vi "Demo UI Orientation.vi"(8 "error in (no error)":errorcluster) -> (0 "error out":errorcluster)   [LabVIEW 2011]
uses:
  VIremote.llb/VIremoteEvent.ctl
  VIremote.llb/VIremoteFunction.ctl
  VIremote.llb/VIremoteStatus.ctl
panel:
  out "Hide":bool
  out "Orientation":T1=enum."Portrait"
  in  "VIremoteEvent":T1=enum."Connection Closed"
  # "Rotate your Device!"
  # "If you have locked your device in one orientation this demo will not work."
  # "This VIs orientation is Landscape"
  # "Portrait"
  # "This VIs orientation is Landscape"
  # "Portrait"
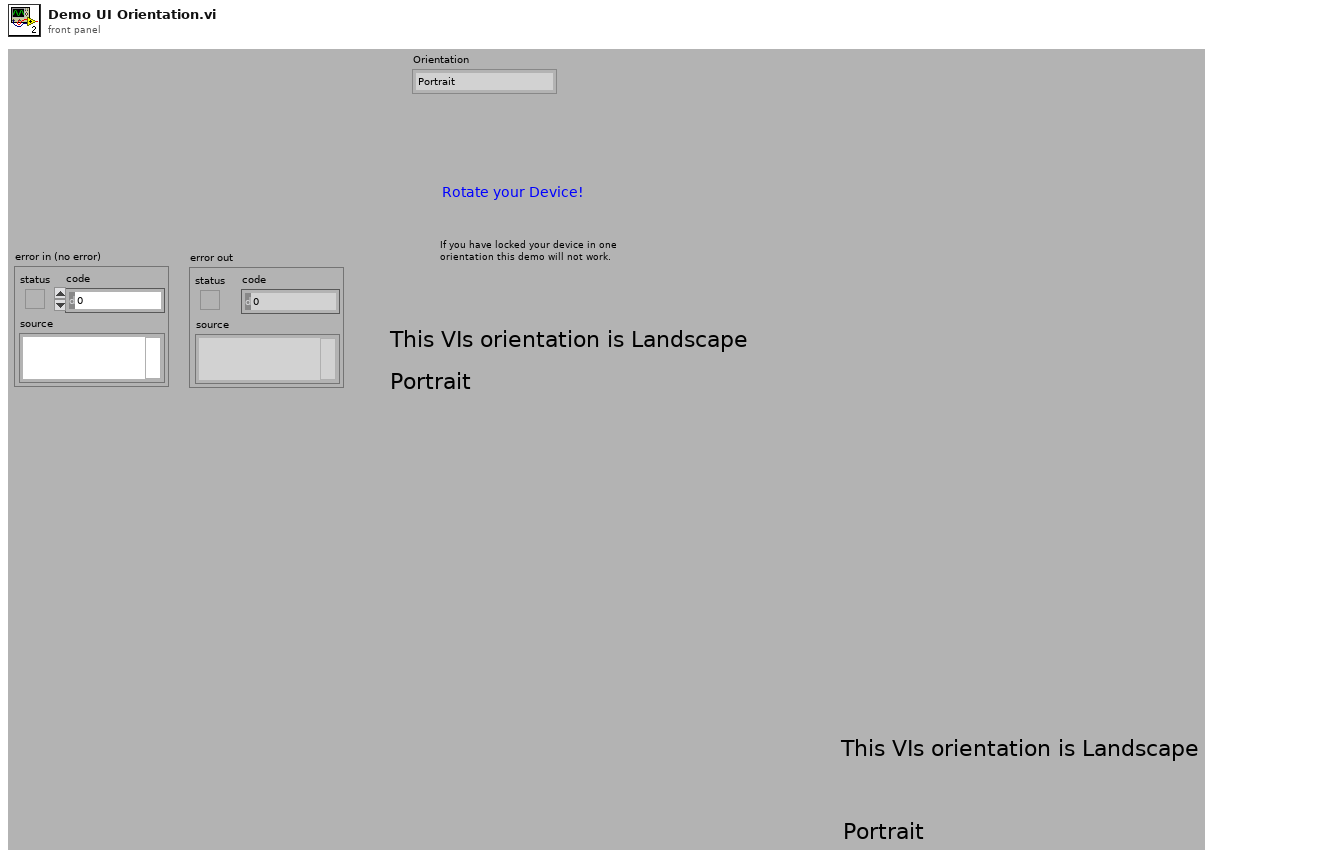
[diagram p1: front panel]
types:
  T1 = typedef "VIremoteEvent.ctl" = enum16{"No Event", "Connection Closed", "Navigate Back", "Enter Background", "Enter Foreground", "Portrait", "Portrait Upside Down", "Landscape Left", "Landscape Right"}
  T2 = typedef "VIremoteStatus.ctl" = enum16{"Connected BOOL", "Number of connections DBL", "VIremoteController ver.", "VIremote ver. DBL", "Screen width DBL", "Screen height DBL", "Current navigation bar height DBL", "Current UI orientation", "Background supported BOOL", "Background state BOOL", "Device UI idiom (0=phone,1=iPad) DBL", "Device name", "Device unique id", "Device system ver.", "Device model", "Device HW model"}
  T3 = typedef "VIremoteFunction.ctl" = enum16{"Do nothing", "Stop controller", "Close this connection", "Show info panel", "Set VI to control", "Set Accelerometer freq (Hz)", "Show Alert message", "Start Sound Input", "Stop Sound Input", "Set Volume (0-100)", "Set sound output Speaker", "Set sound output Receiver", "Play Sound", "Repeat Sound", "Stop Sound", "Pause Sound", "Resume Sound", "Set panel width of caller (320 or 480)", "Set Panel Size to Portrait", "Set Panel Size to Landscape", "Set Panel Size as Current Orientation", "Allow all UI Orientations", "Send user notification", "Disable Scrolling", "Normal Scrolling", "Page Scrolling", "Set Scroll Offset", "Page Indicator Position"}
  T4 = typedef "VIremotePreferences.ctl" = cluster{"Set (must be true)":bool, "allowed UI orientations":cluster{"Portrait":bool, "PortraitUpsideDown":bool, "LandscapeLeft":bool, "LandscapeRight":bool}}
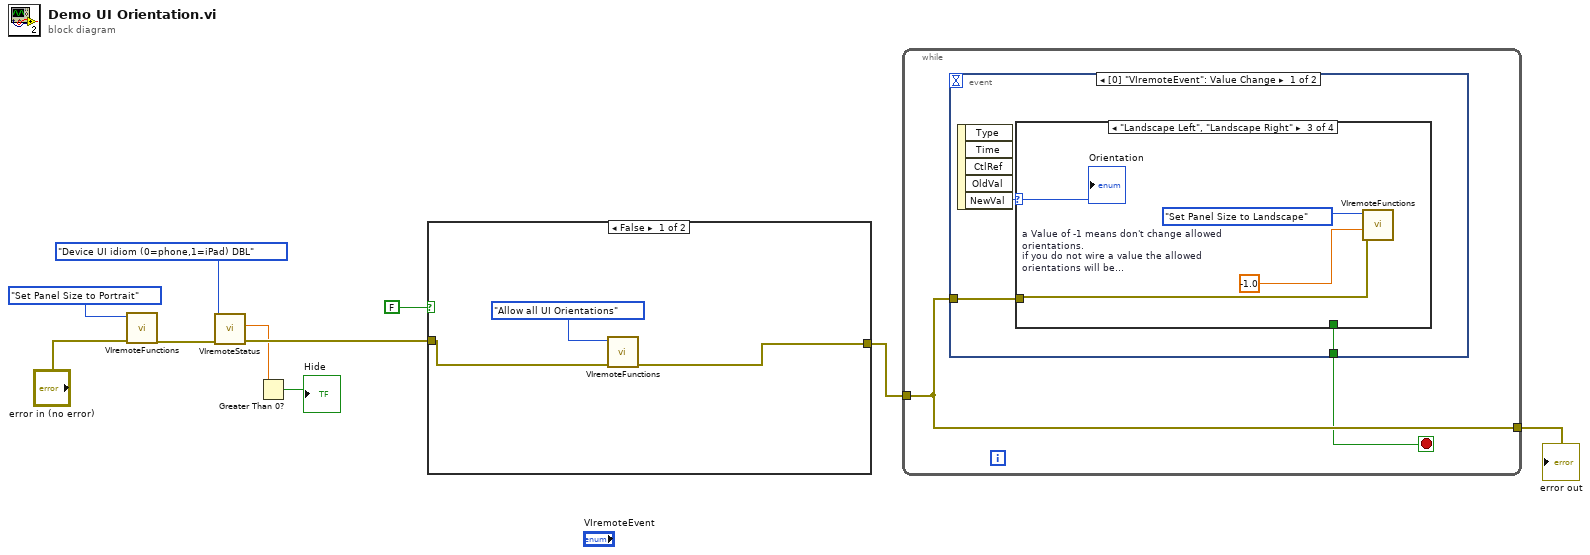
[diagram p0: block diagram]
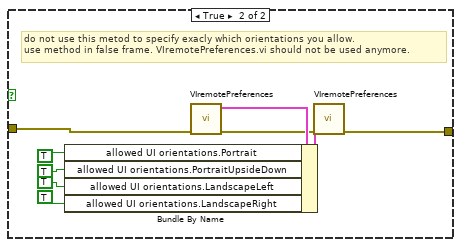
[diagram p2: hidden frame]
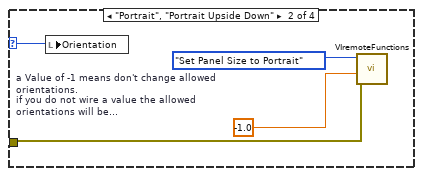
[diagram p4: hidden frame]
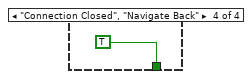
[diagram p5: hidden frame]
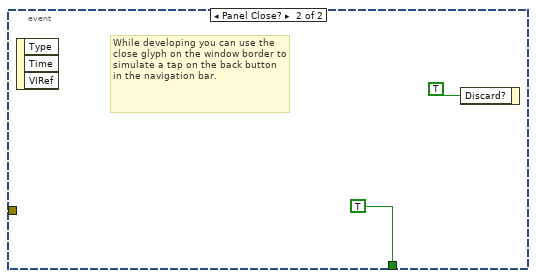
[diagram p6: hidden frame]
diagram:
  n1 = call "VIremoteFunctions.vi"("error in (no error)"="error in (no error)", "Function"=VIremoteFunction."Set Panel Size to Portrait") -> ("error out"=w5:errorcluster)  [unwired: 4 in, 5 out]
  n2 = call "VIremoteStatus.vi"("error in (no error)"=w5, "Status item"=VIremoteStatus."Device UI idiom (0=phone,1=iPad) DBL") -> ("error out"=w4:errorcluster, "DBL"=w2:dbl)  [unwired: 1 in, 7 out]
  n3 = Greater Than 0?(x=w2) -> (x > 0?=→"Hide":bool)
  n4 = case shown="False" FALSE {
    tunnel: [w12 w15] -> w10
    tunnel: w4 -> [w11 w14]
    frame False {
      n5 = call "VIremoteFunctions.vi"("error in (no error)"=w11, "Function"=VIremoteFunction."Allow all UI Orientations") -> ("error out"=w12:errorcluster)  [unwired: 4 in, 5 out]
    }
    frame True {
      # "do not use this metod to specify exacly which orientations you allow.\nuse method in false frame. VIremotePreferences.vi should not be used anymore."
      n6 = call "VIremotePreferences.vi"("error in (no error)"=w14) -> ("error out"=w16:errorcluster, "VIremote Preferences read"=w21:T4)  [unwired: 2 in, 7 out]
      n7 = Bundle By Name(cluster=w21, "allowed UI orientations.Portrait"=TRUE, "allowed UI orientations.PortraitUpsideDown"=TRUE ("allowed UI orientations.Portrait"), "allowed UI orientations.LandscapeLeft"=TRUE ("allowed UI orientations.Portrait"), "allowed UI orientations.LandscapeRight"=TRUE ("allowed UI orientations.Portrait")) -> (w22:T4)
      n8 = call "VIremotePreferences.vi"("error in (no error)"=w16, "VIremote Preferences to set (read)"=w22) -> ("error out"=w15:errorcluster)  [unwired: 1 in, 8 out]
    }
  }
  n9 = while {
    tunnel: w10 -> [w24]
    tunnel: [w24] -> w6
    stop <- w23 stop-if-true
    n10 = event shown="[0] \"VIremoteEvent\": Value Change" {
      selector: _ -> [_ _]
      dyn-events: _ -> [_ _]
      timeout: _ -> [_ _]
      tunnel: w24 -> [w27 _]
      tunnel: [w25 TRUE ("Discard?")] -> w23
      event Value Change {
        n11 = event-data() -> ("NewVal"=w26:T1)  [unwired: 5 out]
        n12 = case shown="\"Landscape Left\", \"Landscape Right\"" w26 {
          selector: w26 -> [_ w28 w32 _]
          tunnel: w27 -> [_ w31 w35 _]
          tunnel: [_ _ _ TRUE] -> w25
          frame "No Event", Default {
          }
          frame "Portrait", "Portrait Upside Down" {
            w30 = -1.0  # a Value of -1 means don't change allowed orientations. if you do not wire a value the allowed orientations will be all landscapes or all portrait orientations.
            n13 = local write "Orientation"(w28) -> ()
            n14 = call "VIremoteFunctions.vi"("error in (no error)"=w31, "Value in"=w30, "Function"=VIremoteFunction."Set Panel Size to Portrait") -> ()  [unwired: 3 in, 6 out]
          }
          frame "Landscape Left", "Landscape Right" {
            w34 = -1.0  # a Value of -1 means don't change allowed orientations. if you do not wire a value the allowed orientations will be all landscapes or all portrait orientations.
            n15 = call "VIremoteFunctions.vi"("error in (no error)"=w35, "Value in"=w34, "Function"=VIremoteFunction."Set Panel Size to Landscape") -> ()  [unwired: 3 in, 6 out]
            "Orientation" <- w32
          }
          frame "Connection Closed", "Navigate Back" {
          }
        }
      }
      event Panel Close? {
        # "While developing you can use the close glyph on the window border to simulate a tap on the back button in the navigation bar."
        n16 = event-data() -> ()  [unwired: 4 out]
        n17 = event-data("Discard?"=TRUE) -> ()  [unwired: 1 in, 1 out]
      }
    }
  }
  "error out" <- w6
